vi "globalSetUp.vi"(8 "error in (no error)":errorcluster, 11 "testcase-CSMResponse in":refnum<class "testcase-CSMResponse.lvclass">) -> (0 "error out":errorcluster, 3 "testcase-CSMResponse out":refnum<class "testcase-CSMResponse.lvclass">)   [LabVIEW 2017, in "testcase-CSMResponse.lvclass"]
uses:
  testcase-CSMResponse.lvclass
  <vilib>/addons/_JKI Toolkits/VI Tester/TestCase.llb/TestCase.lvclass
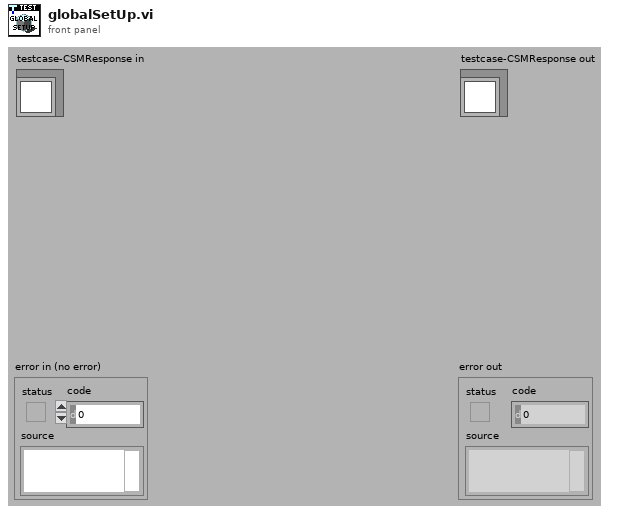
[diagram p1: front panel]
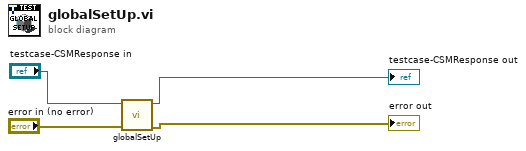
[diagram p0: block diagram]
diagram:
  n1 = call-parent "globalSetUp.vi"("error in (no error)"="error in (no error)", "TestCase in"="testcase-CSMResponse in") -> ("error out"=→"error out":errorcluster, "TestCase out"=→"testcase-CSMResponse out":refnum<class "testcase-CSMResponse.lvclass">)  [unwired: 8 in]
